vi "Handle CHALLENGE.vi"(8 "error in (no error)":errorcluster, 9 "WAMP Message":T1 {"Message Codes" items=["HELLO"=1, "WELCOME"=2, "ABORT"=3, "GOODBYE"=6, "ERROR"=8, "PUBLISH"=16, "PUBLISHED"=17, "SUBSCRIBE"=32, "SUBSCRIBED"=33, "UNSUBSCRIBE"=34, "UNSUBSCRIBED"=35, "EVENT"=36, "CALL"=48, "RESULT"=59, "REGISTER"=64, "REGISTERED"=65, "UNREGISTER"=66, "UNREGISTERED"=67, "INVOCATION"=68, "YIELD"=70]}, 11 "WAMP Client in":refnum<class "WAMP Client.lvclass">) -> (0 "error out":errorcluster, 1 "Response":string, 3 "WAMP Client out":refnum<class "WAMP Client.lvclass">)   [LabVIEW 2020, in "wamplv.lvlib" / "WAMP Client.lvclass"]
uses:
  WAMP Client.lvclass
  TypeDef/WAMP Received Message.ctl
  TypeDef/WAMP Message Codes.ctl
  WAMP Client.lvclass/WAMP Client.ctl
  36fadca6-ec9a-4dfa-8a83-2e68193b1adb.vi
  <vilib>/JDP Science/JSONtext/JSON text to Variant.vi
  <vilib>/Utility/error.llb/Error Cluster From Error Code.vi
  <vilib>/JDP Science/JSONtext/LVClass Serializer/JSONtext LVClass Serializer.lvclass
  <vilib>/ErrorRing/Error Ring.xnode
  Private/Authenticators/IAuthenticator/IAuthenticator.lvclass
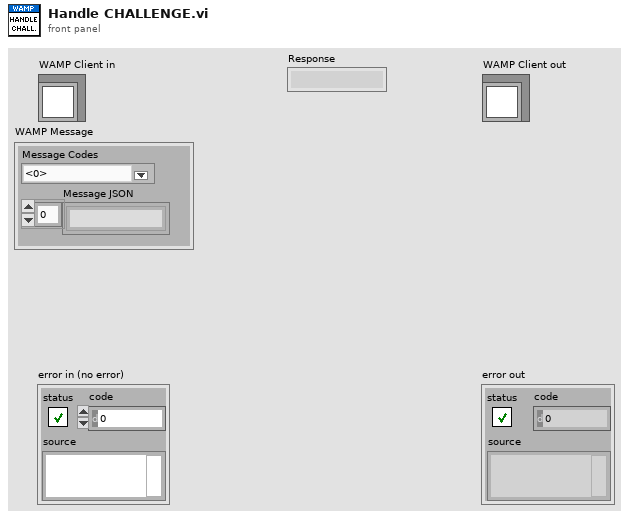
[diagram p1: front panel]
types:
  T1 = typedef "wamplv.lvlib/WAMP Client.lvclass/WAMP Received Message.ctl" = cluster{"Message JSON":string[], "Message Codes":T2}
  T2 = typedef "wamplv.lvlib/WAMP Client.lvclass/WAMP Message Codes.ctl" = u16
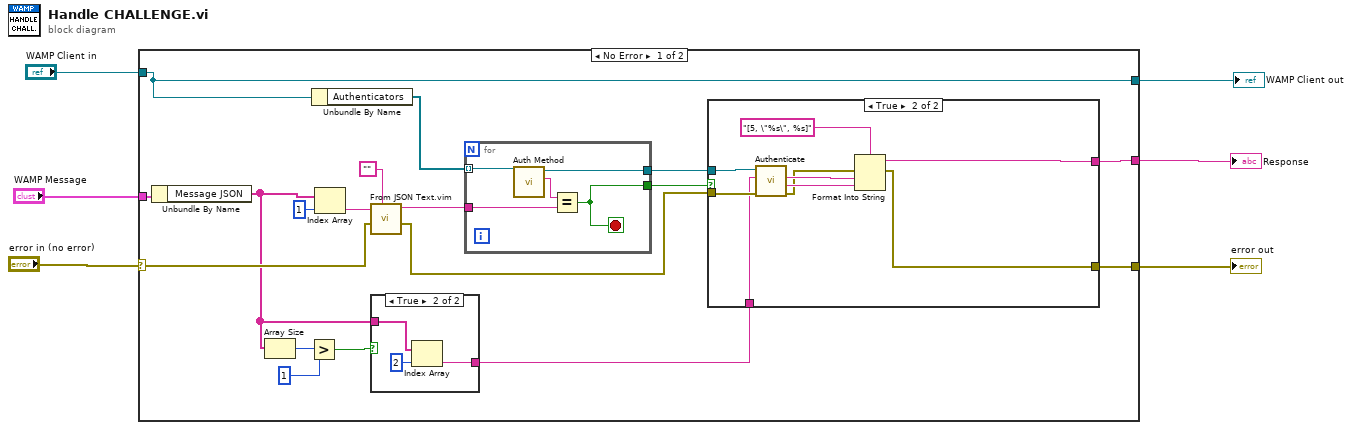
[diagram p0: block diagram]
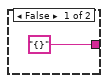
[diagram p2: hidden frame]
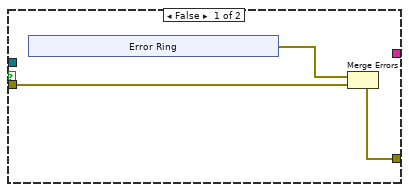
[diagram p3: hidden frame]
diagram:
  n1 = case shown="No Error" "error in (no error)" {
    selector: "error in (no error)" -> [w20 w51]
    tunnel: [w8 w51] -> w5
    tunnel: [w19 w50] -> w3
    tunnel: "WAMP Client in" -> [w19 w50]
    tunnel: "WAMP Message" -> [w24 _]
    tunnel: [w7 _] -> w1
    frame No Error {
      n2 = Unbundle By Name(w24) -> ("Message JSON"=w10:string[])
      n3 = Array Size(array=w10) -> (size(s)=w13:i32)
      n4 = Greater?(x=w13, y=1) -> (0:w11:bool)
      n5 = Unbundle By Name(w19) -> ("Authenticators"=w18:refnum<class "IAuthenticator.lvclass">[])
      n6 = Index Array(array=w10, index=1) -> (element=w22:string)
      n7 = call "From JSON Text.vim"("Data Type and Default Value"="", "error in (no error)"=w20, "JSON"=w22) -> ("error out"=w14:errorcluster, "Data out"=w17:string)  [unwired: 7 in]
      n8 = case shown="True" w11 {
        tunnel: w10 -> [_ w27]
        tunnel: ["{}" ("<JSON>") w26] -> w9
        frame False {
        }
        frame True {
          n9 = Index Array(array=w27, index=2) -> (element=w26:string)
        }
      }
      n10 = for {
        tunnel: w18 -> [w49] mode=indexing
        tunnel: w17 -> [w47]
        tunnel: [w46] -> w16
        tunnel: [w45] -> w15
        stop <- w45 stop-if-true
        n11 = call-dynamic "Auth Method.vi"("IAuthenticator in"=w49) -> ("Authmethod"=w48:string, "IAuthenticator out"=w46:refnum<class "IAuthenticator.lvclass">)  [unwired: 9 in]
        n12 = Equal?(x=w48, y=w47) -> (x = y?=w45:bool)
      }
      n13 = case shown="True" w15 {
        tunnel: w16 -> [_ w44]
        tunnel: w14 -> [w30 w43]
        tunnel: w9 -> [_ w39]
        tunnel: [w29 w37] -> w8
        tunnel: [_ w36] -> w7
        frame False {
          n14 = xnode "Error Ring"() -> ("error out"=w31:errorcluster)
          n15 = Merge Errors(w31, w30) -> (w29:errorcluster)
        }
        frame True {
          n16 = call "Authenticate.vi"("error in (no error)"=w43, "Challenge Dict"=w39, "IAuthenticator in"=w44) -> ("error out"=w38:errorcluster, "Authenticate Dict"=w40:string, "Authenticate Signature"=w41:string)  [unwired: 5 in, 1 out]
          n17 = Format Into String(format string="[5, \"%s\", %s]", error in=w38, w41, w40) -> (resulting string=w36:string, error out=w37:errorcluster)  [unwired: 1 in]
        }
      }
    }
    frame Error {
    }
  }
  "error out" <- w5
  "WAMP Client out" <- w3
  "Response" <- w1
